vi "_PC_Pub_FM setMachineType.vi"(8 "error in (no error)":errorcluster, 11 "FM in":refnum<class "FM.lvclass">) -> (0 "error out":errorcluster, 3 "FM out":refnum<class "FM.lvclass">)   [LabVIEW 2018, in "FM.lvclass"]
uses:
  FM.lvclass
  DataXML/DataXML.lvclass
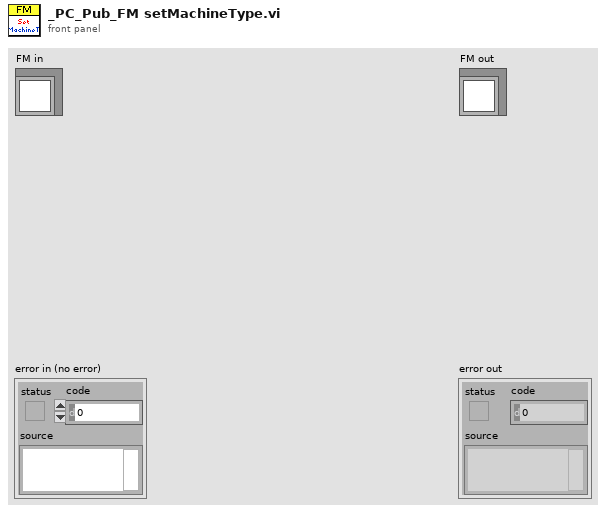
[diagram p1: front panel]
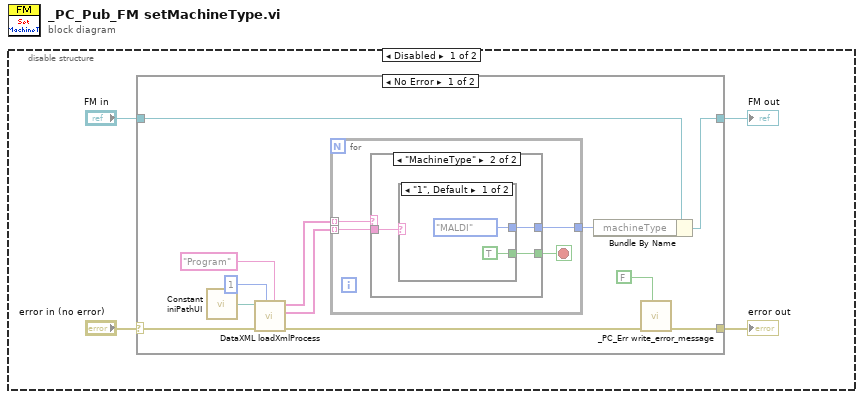
[diagram p0: block diagram]
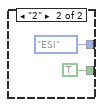
[diagram p3: hidden frame]
diagram:
  n1 = disable-structure shown="Disabled" {
    frame Disabled {
      n2 = case shown="No Error" "error in (no error)" {
        selector: "error in (no error)" -> [w8 w29]
        tunnel: [w5 w29] -> w3
        tunnel: [w15 w28] -> w1
        tunnel: "FM in" -> [w16 w28]
        frame No Error {
          n3 = call "Constant iniPathUI.vi"() -> ("appended path"=w10:path)
          n4 = call "DataXML loadXmlProcess.vi"("target name"="Program", "level"=u8 1, "error in (no error)"=w8, "xml_data_path"=w10) -> ("error IO"=w6:errorcluster, "value"=w14:string[], "name"=w13:string[])  [unwired: 4 in, 1 out]
          n5 = for {
            tunnel: w13 -> [w20] mode=indexing
            tunnel: w14 -> [w19] mode=indexing
            tunnel: [w18] -> w9
            stop <- w17 stop-if-true
            n6 = case shown="\"MachineType\"" w20 {
              tunnel: w19 -> [_ w23]
              tunnel: [_ w22] -> w18
              tunnel: [_ w21] -> w17
              frame Default {
              }
              frame "MachineType" {
                n7 = case shown="\"1\", Default" w23 {
                  tunnel: [enum16{"MALDI", "ESI"}."MALDI" ("machineType") enum16{"MALDI", "ESI"}."ESI" ("machineType")] -> w22
                  tunnel: [TRUE TRUE] -> w21
                  frame "1", Default {
                  }
                  frame "2" {
                  }
                }
              }
            }
          }
          n8 = Bundle By Name(cluster=w16, "machineType"=w9) -> (w15:refnum<class "FM.lvclass">)
          n9 = call "_PC_Err write_error_message.vi"("show msg( T )"=FALSE, "error in"=w6) -> ("error out"=w5:errorcluster)  [unwired: 9 in]
        }
        frame Error {
        }
      }
      "error out" <- w3
      "FM out" <- w1
    }
    frame Enabled {
    }
  }
